vi "SMO.Control Experiment.Command Enum to String.vi"(8 "error in (no error)":errorcluster, 10 "Commands":T1, 11 "Control Experiment":refnum<class "SMO.Control Experiment.lvclass">) -> (0 "error out":errorcluster, 1 "Commands []":string[](array[string]), 2 "Command":string, 3 "Control Experiment out":refnum<class "SMO.Control Experiment.lvclass">)   [LabVIEW 2019, in "SMO.Control Experiment.lvclass"]
uses:
  SMO.Control Experiment.lvclass
  Typedefs/SMO.Control Experiment.Commands--Enum.ctl
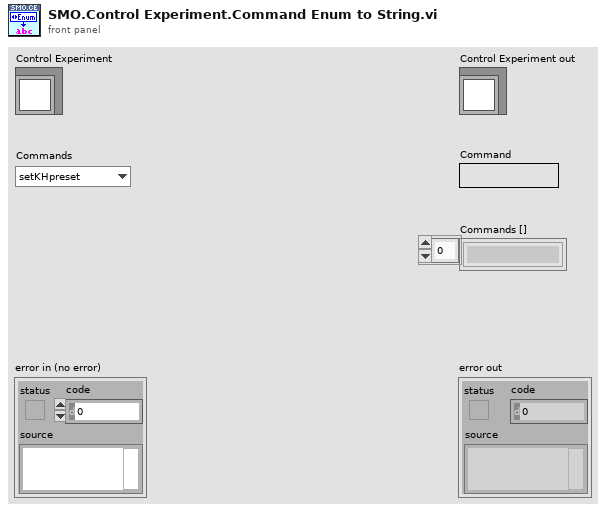
[diagram p1: front panel]
types:
  T1 = typedef "SMO.Control Experiment.lvclass/SMO.Control Experiment.Commands--Enum.ctl" = enum16{"setKHpreset", "getXML", "saveData"}
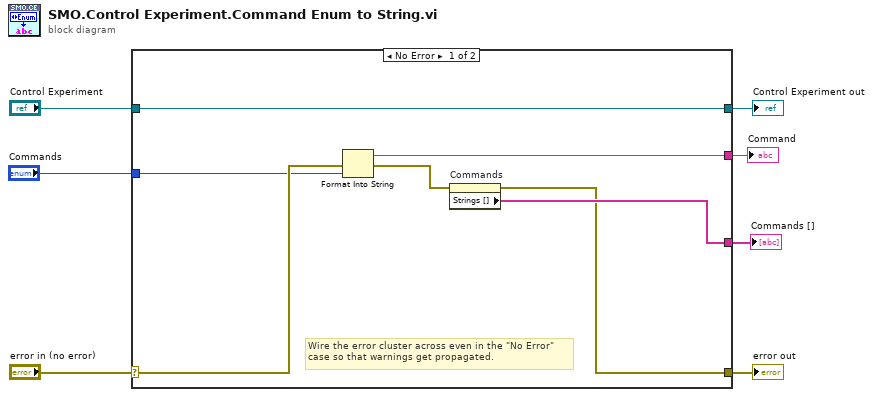
[diagram p0: block diagram]
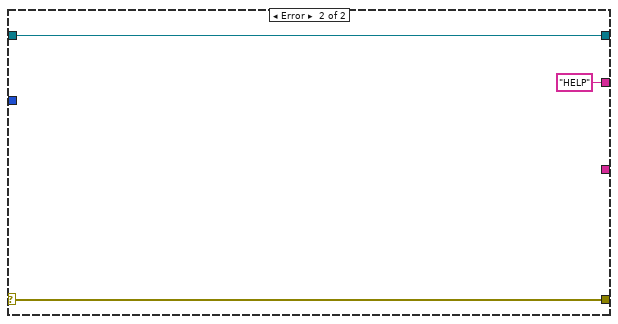
[diagram p2: hidden frame]
diagram:
  n1 = case shown="No Error" "error in (no error)" {
    selector: "error in (no error)" -> [w13 w17]
    tunnel: [w8 w17] -> w6
    tunnel: [w14 w16] -> w4
    tunnel: "Control Experiment" -> [w14 w16]
    tunnel: "Commands" -> [w12 _]
    tunnel: [w11 "HELP"] -> w2
    tunnel: [w10 _] -> w1
    frame No Error {
      # "Wire the error cluster across even in the \"No Error\"\ncase so that warnings get propagated."
      n2 = Format Into String(error in=w13, w12) -> (resulting string=w11:string, error out=w9:errorcluster)  [unwired: 2 in]
      n3 = property on="Commands" class="Enum (strict)"(error in=w9) -> (error out=w8:errorcluster, "Strings []"=w10:string[])  [unwired: 1 in, 1 out]
    }
    frame Error {
    }
  }
  "error out" <- w6
  "Control Experiment out" <- w4
  "Command" <- w2
  "Commands []" <- w1
